vi "PostUUT.vi"(8 "error in (no error)":errorcluster, 10 "Execution in":refnum<data-value>, 11 "TestProjectBase in":refnum<class "Project.lvclass">) -> (0 "error out":errorcluster, 2 "Execution out":refnum<data-value>, 3 "TestProjectBase out":refnum<class "Project.lvclass">)   [LabVIEW 2015, in "Project.lvclass"]
uses:
  Project.lvclass
  Execution.lvclass
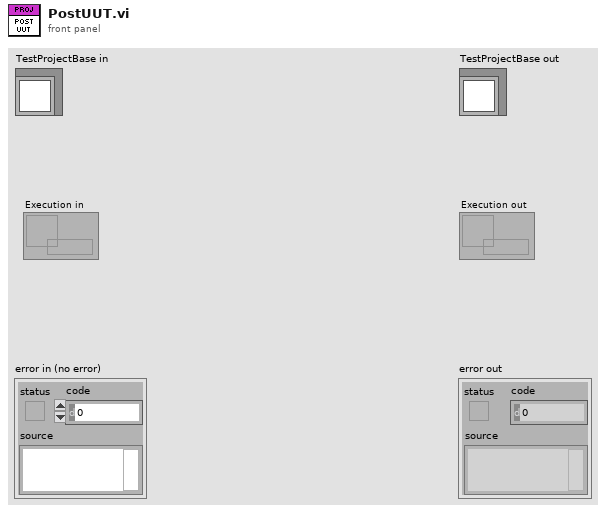
[diagram p1: front panel]
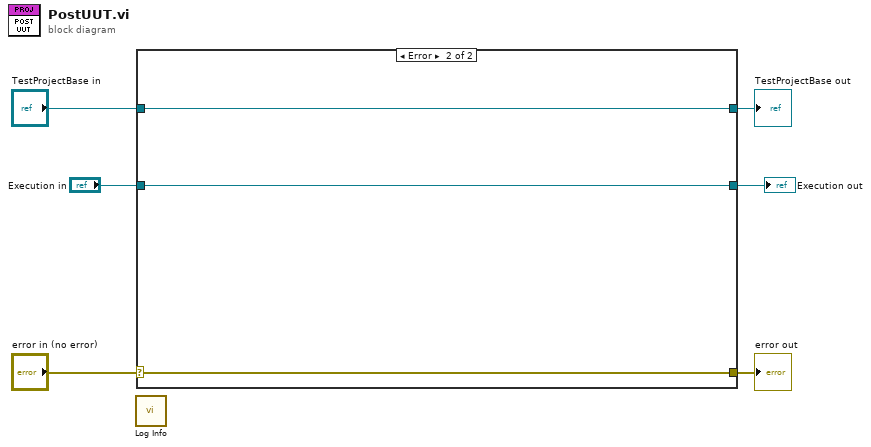
[diagram p0: block diagram]
diagram:
  n1 = call "Log Info.vi"() -> ()  [unwired: 5 in, 1 out]
  n2 = case shown="Error" "error in (no error)" {
    selector: "error in (no error)" -> [w8 w12]
    tunnel: [w8 w12] -> w5
    tunnel: [w9 w11] -> w3
    tunnel: "TestProjectBase in" -> [w9 w11]
    tunnel: "Execution in" -> [w7 w10]
    tunnel: [w7 w10] -> w1
    frame No Error {
    }
    frame Error {
    }
  }
  "error out" <- w5
  "TestProjectBase out" <- w3
  "Execution out" <- w1
